vi "PrintGraph (SubVI).vi"(6 "AFR,EGT-Graph Ref":refnum<vi>, 7 "AFR, EGT":bool, 8 "Überschrift":refnum<vi>, 9 "Ergebnis":refnum<vi>, 10 "Fahrzeugdaten":refnum<vi>, 11 "P+M Graph Ref":refnum<vi>) -> ()   [LabVIEW 2014]
uses:
  <vilib>/Utility/NIReport.llb/HTML Report Image Alignment.ctl
  <vilib>/Utility/NIReport.llb/Append Report Text (str wrap).vi
  <vilib>/Utility/NIReport.llb/NI_report.lvclass
  <vilib>/Utility/NIReport.llb/NI_ReportGenerationCore.lvlib
panel:
  out "AFR,EGT-Graph":cluster{dbl[], dbl[]}[](graph)
  out "P+M Graph":cluster{dbl[], dbl[]}[](graph) caption="XY-Graph"
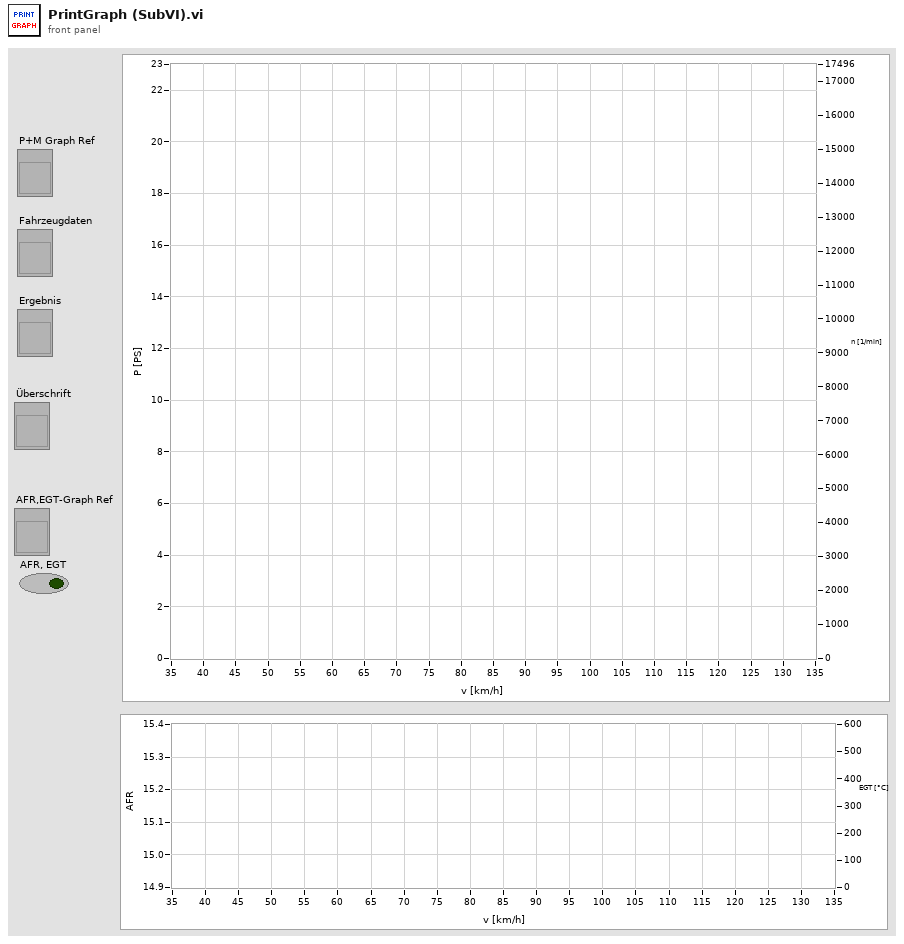
[diagram p1: front panel]
types:
  T1 = cluster{"Charset (-1)":i16, "Weight (-1)":i16, "Name":string, "Size":string}
  T2 = cluster{"Italic":enum16{"Italic Unchanged", "Italic On", "Italic Off"}, "Strike Through":enum16{"Strike Through Unchanged", "Strike Through On", "Strike Through Off"}, "Underline":enum16{"Underline Unchanged", "Underline On", "Underline Off"}, "Bold":enum16{"Bold Unchanged", "Bold On", "Bold Off"}}
  T3 = typedef "LVRangeTypeDef.ctl" = cluster{"Minimum":dbl, "Maximum":dbl, "Increment":dbl, "Minor Increment":dbl, "Start":dbl}
  T4 = typedef "NI_ReportGenerationCore.lvlib/HTML Report Image Alignment.ctl" = enum16{"(default)", "LEFT", "RIGHT", "TOP", "TEXTTOP", "MIDDLE", "ABSMIDDLE", "BASELINE", "BOTTOM", "ABSBOTTOM"}
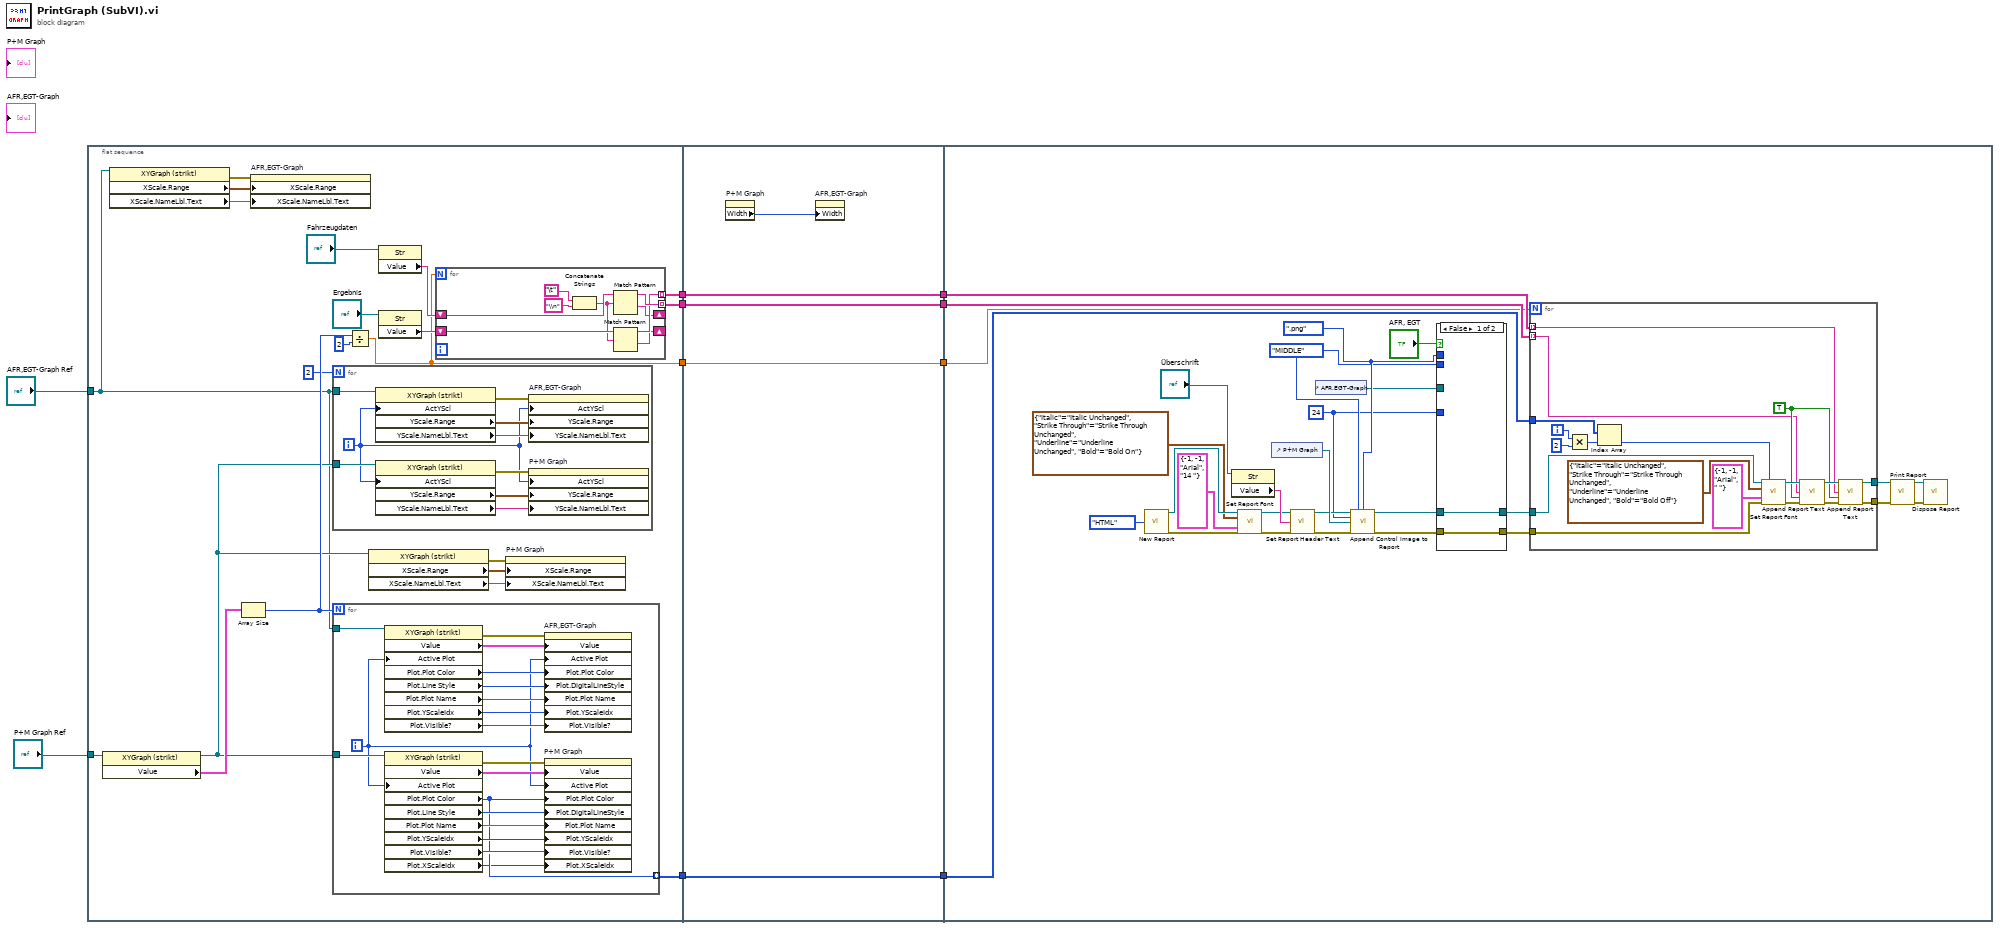
[diagram p0: block diagram]
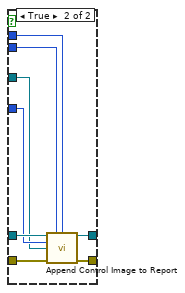
[diagram p2: hidden frame]
diagram:
  n1 = flat-sequence {
    tunnel: "P+M Graph Ref" -> [w31]
    tunnel: [w27] -> w8
    tunnel: [w24] -> w6
    tunnel: [w23] -> w4
    tunnel: [w21] -> w2
    tunnel: "AFR,EGT-Graph Ref" -> [w11]
    tunnel: w8 -> [w72]
    tunnel: [w72] -> w7
    tunnel: w6 -> [w71]
    tunnel: [w71] -> w5
    tunnel: w4 -> [w70]
    tunnel: [w70] -> w3
    tunnel: w2 -> [w69]
    tunnel: [w69] -> w1
    tunnel: w7 -> [w95]
    tunnel: w5 -> [w94]
    tunnel: w3 -> [w93]
    tunnel: w1 -> [w92]
    frame #0 {
      n2 = property on="Eigenschaftsknoten" class="XYGraph (strikt)"(reference=w31) -> (reference out=w18:refnum<vi>, "Value"=w30:cluster{dbl[], dbl[]}[])  [unwired: 1 in, 1 out]
      n3 = property on="Eigenschaftsknoten" class="XYGraph (strikt)"(reference=w11) -> (error out=w13:errorcluster, "XScale.Range"=w12:T3, "XScale.NameLbl.Text"=w14:string)  [unwired: 1 in, 1 out]
      n4 = Array Size(array=w30) -> (size(s)=w20:i32)
      n5 = property on="AFR,EGT-Graph" class="XYGraph (strikt)"(error in=w13, "XScale.Range"=w12, "XScale.NameLbl.Text"=w14) -> ()  [unwired: 1 in, 2 out]
      n6 = for {
        N: 2 -> [_]
        tunnel: w18 -> [w48]
        tunnel: w11 -> [w42]
        i -> [w41]
        n7 = property on="Eigenschaftsknoten" class="XYGraph (strikt)"(reference=w42, "ActYScl"=w41) -> (error out=w45:errorcluster, "YScale.Range"=w43:T3, "YScale.NameLbl.Text"=w44:string)  [unwired: 1 in, 1 out]
        n8 = property on="Eigenschaftsknoten" class="XYGraph (strikt)"(reference=w48, "ActYScl"=w41) -> (error out=w46:errorcluster, "YScale.Range"=w49:T3, "YScale.NameLbl.Text"=w47:string)  [unwired: 1 in, 1 out]
        n9 = property on="AFR,EGT-Graph" class="XYGraph (strikt)"(error in=w45, "ActYScl"=w41, "YScale.Range"=w43, "YScale.NameLbl.Text"=w44) -> ()  [unwired: 1 in, 2 out]
        n10 = property on="P+M Graph" class="XYGraph (strikt)"(error in=w46, "ActYScl"=w41, "YScale.Range"=w49, "YScale.NameLbl.Text"=w47) -> ()  [unwired: 1 in, 2 out]
      }
      n11 = for {
        N: w20 -> [_]
        tunnel: w18 -> [w64]
        tunnel: [w60] -> w27 mode=indexing
        tunnel: w11 -> [w50]
        i -> [w51]
        n12 = property on="Eigenschaftsknoten" class="XYGraph (strikt)"(reference=w50, "Active Plot"=w51) -> (error out=w57:errorcluster, "Value"=w56:cluster{dbl[], dbl[]}[], "Plot.Plot Color"=w58:u32, "Plot.Line Style"=w52:u8, "Plot.Plot Name"=w53:string, "Plot.YScaleIdx"=w54:u32, "Plot.Visible?"=w55:bool)  [unwired: 1 in, 1 out]
        n13 = property on="Eigenschaftsknoten" class="XYGraph (strikt)"(reference=w64, "Active Plot"=w51) -> (error out=w61:errorcluster, "Value"=w62:cluster{dbl[], dbl[]}[], "Plot.Plot Color"=w60:u32, "Plot.Line Style"=w67:u8, "Plot.Plot Name"=w66:string, "Plot.YScaleIdx"=w65:u32, "Plot.Visible?"=w63:bool, "Plot.XScaleIdx"=w59:u32)  [unwired: 1 in, 1 out]
        n14 = property on="AFR,EGT-Graph" class="XYGraph (strikt)"(error in=w57, "Value"=w56, "Active Plot"=w51, "Plot.Plot Color"=w58, "Plot.DigitalLineStyle"=w52, "Plot.Plot Name"=w53, "Plot.YScaleIdx"=w54, "Plot.Visible?"=w55) -> ()  [unwired: 1 in, 2 out]
        n15 = property on="P+M Graph" class="XYGraph (strikt)"(error in=w61, "Value"=w62, "Active Plot"=w51, "Plot.Plot Color"=w60, "Plot.DigitalLineStyle"=w67, "Plot.Plot Name"=w66, "Plot.YScaleIdx"=w65, "Plot.Visible?"=w63, "Plot.XScaleIdx"=w59) -> ()  [unwired: 1 in, 2 out]
      }
      n16 = Divide(x=w20, y=u32 2) -> (x/y=w21:dbl)
      n17 = property on="Eigenschaftsknoten" class="XYGraph (strikt)"(reference=w18) -> (error out=w17:errorcluster, "XScale.Range"=w19:T3, "XScale.NameLbl.Text"=w16:string)  [unwired: 1 in, 1 out]
      n18 = property class="Str"(reference="Fahrzeugdaten") -> ("Value"=w25:string)  [unwired: 1 in, 2 out]
      n19 = property class="Str"(reference="Ergebnis") -> ("Value"=w26:string)  [unwired: 1 in, 2 out]
      n20 = for {
        N: w21 -> [_]
        tunnel: [w37] -> w24 mode=indexing
        tunnel: [w38] -> w23 mode=indexing
        shift-right: [w34] -> _
        shift-left: w26 -> [w40]
        shift-right: [w33] -> _
        shift-left: w25 -> [w39]
        n21 = Concatenate Strings("\t", "\\n" ("Regulärer Ausdruck")) -> (w36:string)
        n22 = Match Pattern(string=w39, regular expression=w36) -> (before substring=w38:string, after substring=w33:string)  [unwired: 1 in, 2 out]
        n23 = Match Pattern(string=w40, regular expression=w36) -> (before substring=w37:string, after substring=w34:string)  [unwired: 1 in, 2 out]
      }
      n24 = property on="P+M Graph" class="XYGraph (strikt)"(error in=w17, "XScale.Range"=w19, "XScale.NameLbl.Text"=w16) -> ()  [unwired: 1 in, 2 out]
    }
    frame #1 {
      n25 = property on="P+M Graph" class="XYGraph (strikt)"() -> ("Width"=w68:u32)  [unwired: 2 in, 2 out]
      n26 = property on="AFR,EGT-Graph" class="XYGraph (strikt)"("Width"=w68) -> ()  [unwired: 2 in, 2 out]
    }
    frame #2 {
      w76 = HTML_Report_Image_Alignment."MIDDLE" ("alignment (default)")
      w77 = enum16{".jpg", ".png"}.".png" ("image file type (.jpg)")
      w75 = 24
      n27 = call <vilib>:"New Report.vi"("report type"=enum16{"Standard Report", "HTML"}."HTML") -> ("report out"=w87:refnum<class "NI_report.lvclass">, "error out"=w86:errorcluster)  [unwired: 13 in]
      n28 = property on="Eigenschaftsknoten" class="Str"(reference="Überschrift") -> ("Value"=w88:string)  [unwired: 1 in, 2 out]
      n29 = call-dynamic "Set Report Font.vi"("report in"=w87, "text options"=T2 {"Italic"=enum."Italic Unchanged", "Strike Through"=enum."Strike Through Unchanged", "Underline"=enum."Underline Unchanged", "Bold"=enum."Bold On"}, "font settings"=T1 {"Charset (-1)"=-1, "Weight (-1)"=-1, "Name"="Arial", "Size"="14 "}, "error in (no error)"=w86) -> ("report out"=w84:refnum<class "NI_report.lvclass">, "error out"=w85:errorcluster)  [unwired: 9 in, 1 out]
      n30 = control-ref of="P+M Graph"() -> (w98:refnum<vi>)
      n31 = call-dynamic "Set Report Header Text.vi"("report in"=w84, "center header text"=w88, "error in (no error)"=w85) -> ("report out"=w90:refnum<class "NI_report.lvclass">, "error out"=w91:errorcluster)  [unwired: 11 in]
      n32 = control-ref of="AFR,EGT-Graph"() -> (w74:refnum<vi>)
      n33 = call-dynamic "Append Control Image to Report.vi"("report in"=w90, "alignment (default)"=w76, "image file type (.jpg)"=w77, "image depth"=w75, "ctrl reference"=w98, "error in (no error)"=w91) -> ("report out"=w81:refnum<class "NI_report.lvclass">, "error out"=w79:errorcluster)  [unwired: 6 in, 2 out]
      n34 = case shown="False" "AFR, EGT" {
        tunnel: w81 -> [w103 w111]
        tunnel: [w103 w110] -> w80
        tunnel: w79 -> [w102 w109]
        tunnel: [w102 w108] -> w78
        tunnel: w77 -> [_ w107]
        tunnel: w76 -> [_ w106]
        tunnel: w75 -> [_ w105]
        tunnel: w74 -> [_ w104]
        frame False {
        }
        frame True {
          n35 = call-dynamic "Append Control Image to Report.vi"("report in"=w111, "alignment (default)"=w106, "image file type (.jpg)"=w107, "image depth"=w105, "ctrl reference"=w104, "error in (no error)"=w109) -> ("report out"=w110:refnum<class "NI_report.lvclass">, "error out"=w108:errorcluster)  [unwired: 6 in, 2 out]
        }
      }
      n36 = for {
        N: w92 -> [_]
        tunnel: w78 -> [w127]
        tunnel: [w122] -> w96
        tunnel: w80 -> [w129]
        tunnel: [w123] -> w97
        tunnel: w95 -> [w120]
        tunnel: w94 -> [w115] mode=indexing
        tunnel: w93 -> [w114] mode=indexing
        i -> [w118]
        w121 = TRUE
        n37 = Multiply(x=w118, y=2) -> (x*y=w119:i32)
        n38 = Index Array(array=w120, index=w119) -> (element=w116:u32)
        n39 = call-dynamic "Set Report Font.vi"("report in"=w129, "text color (unchanged)"=w116, "text options"=T2 {"Italic"=enum."Italic Unchanged", "Strike Through"=enum."Strike Through Unchanged", "Underline"=enum."Underline Unchanged", "Bold"=enum."Bold Off"}, "font settings"=T1 {"Charset (-1)"=-1, "Weight (-1)"=-1, "Name"="Arial", "Size"=" "}, "error in (no error)"=w127) -> ("report out"=w128:refnum<class "NI_report.lvclass">, "error out"=w126:errorcluster)  [unwired: 8 in, 1 out]
        n40 = call-poly <vilib>:"Append Report Text.vi"("report in"=w128, "text"=w114, "append on new line? (F)"=w121, "error in (no error)"=w126) -> ("report out"=w125:refnum<class "NI_report.lvclass">, "error out"=w124:errorcluster)  [unwired: 8 in, 2 out]
        n41 = call-poly <vilib>:"Append Report Text.vi"("report in"=w125, "text"=w115, "append on new line? (F)"=w121, "error in (no error)"=w124) -> ("report out"=w123:refnum<class "NI_report.lvclass">, "error out"=w122:errorcluster)  [unwired: 8 in, 2 out]
      }
      n42 = call-dynamic "Print Report.vi"("report in"=w97, "error in (no error)"=w96) -> ("report out"=w100:refnum<class "NI_report.lvclass">, "error out"=w101:errorcluster)  [unwired: 12 in]
      n43 = call-dynamic "Dispose Report.vi"("report in"=w100, "error in (no error)"=w101) -> ()  [unwired: 13 in, 1 out]
    }
  }
